vi "go to angle.vi"(6 "Pause Time [ms]":i32=50, 8 "error in (no error)":errorcluster, 9 "Velocity [rpm]":i32=5, 10 "Angle":dbl, 11 "CL57RS in":refnum<class "CL57RS.lvclass">) -> (0 "error out":errorcluster, 3 "CL57RS out":refnum<class "CL57RS.lvclass">)   [LabVIEW 2025, in "Motor.lvlib" / "CL57RS.lvclass"]
uses:
  CL57RS.lvclass
  CL57RS.lvclass/CL57RS.ctl
  Stepper/Path Mode.ctl
  Motor.lvlib
panel:
  out "Running?":bool
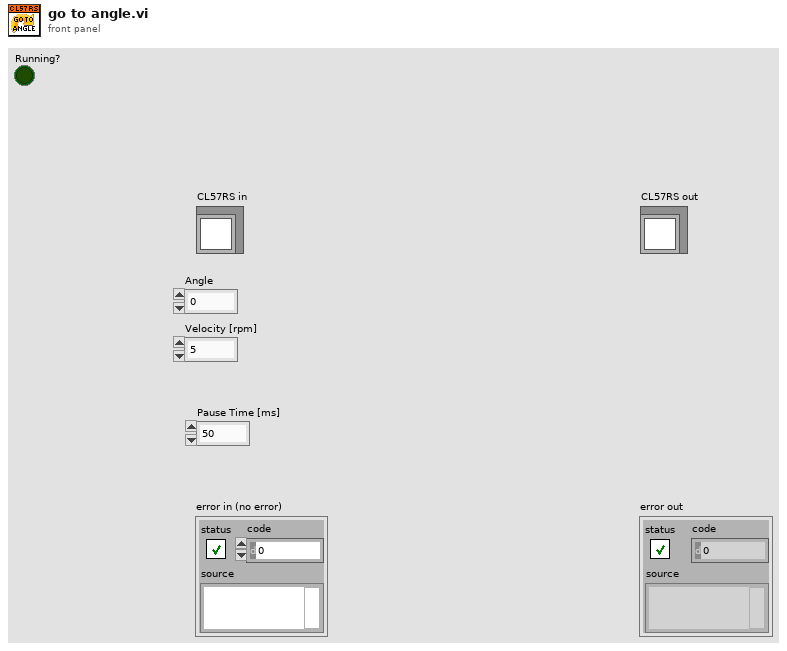
[diagram p1: front panel]
types:
  T1 = typedef "Motor.lvlib/Path Mode.ctl" = enum16{"Position Mode", "Velocity Mode", "Homing Mode"}
  T2 = cluster{"Path Number":i32, "Path Mode":T1, "Relative?":enum16{"Relative", "Absolute"}, "Angle":dbl, "Velocity [rpm]":i32, "Acceleration [ms/krpm]":i32, "Deceleration [ms/krpm]":i32, "Pause Time [ms]":i32}
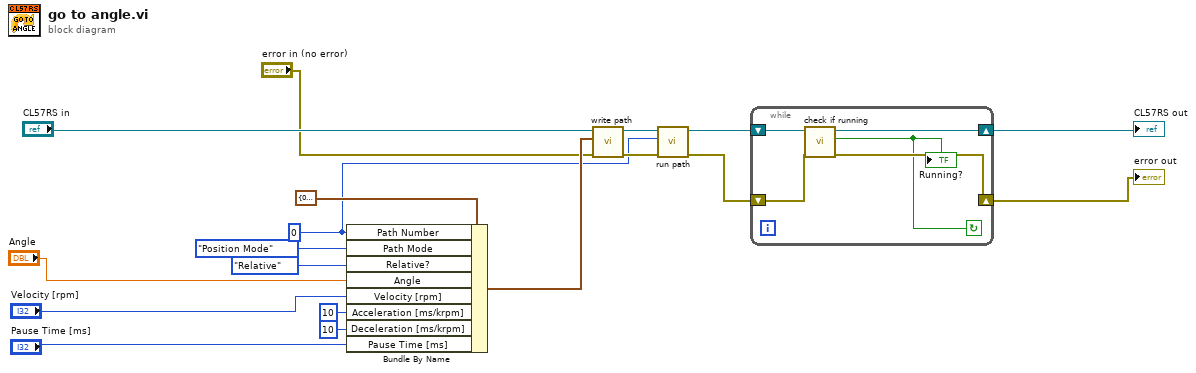
[diagram p0: block diagram]
diagram:
  w10 = 0 ("Path Number")
  n1 = Bundle By Name(cluster=T2 {"Path Number"=0, "Path Mode"=enum."Position Mode", "Relative?"=enum."Relative", "Angle"=0.0, "Velocity [rpm]"=0, "Acceleration [ms/krpm]"=0, "Deceleration [ms/krpm]"=0, "Pause Time [ms]"=0} ("Path Cluster"), "Path Number"=w10, "Path Mode"=Path_Mode."Position Mode", "Relative?"=enum16{"Relative", "Absolute"}."Relative", "Angle"="Angle", "Velocity [rpm]"="Velocity [rpm]", "Acceleration [ms/krpm]"=10, "Deceleration [ms/krpm]"=10, "Pause Time [ms]"="Pause Time [ms]") -> (w12:T2)
  n2 = call "write path.vi"("error in (no error)"="error in (no error)", "Path Cluster"=w12, "CL57RS in"="CL57RS in") -> ("error out"=w11:errorcluster, "CL57RS out"=w18:refnum<class "CL57RS.lvclass">)  [unwired: 7 in]
  n3 = call "run path.vi"("error in (no error)"=w11, "Path Number"=w10, "CL57RS in"=w18) -> ("error out"=w8:errorcluster, "CL57RS out"=w9:refnum<class "CL57RS.lvclass">)  [unwired: 7 in]
  n4 = while {
    shift-right: [w23] -> w7
    shift-left: w9 -> [w22]
    shift-right: [w20] -> w1
    shift-left: w8 -> [w21]
    stop <- w19 continue-if-true
    n5 = call-dynamic "check if running.vi"("error in (no error)"=w21, "CL57RS in"=w22) -> ("error out"=w20:errorcluster, "Running?"=w19:bool, "CL57RS out"=w23:refnum<class "CL57RS.lvclass">)  [unwired: 7 in]
    "Running?" <- w19
  }
  "error out" <- w1
  "CL57RS out" <- w7
